vi "Set Maximum Data Length.vi"(9 "maximum data length":i32=-1, 11 "variant in":variant) -> (3 "variant out":variant)   [LabVIEW 2017]
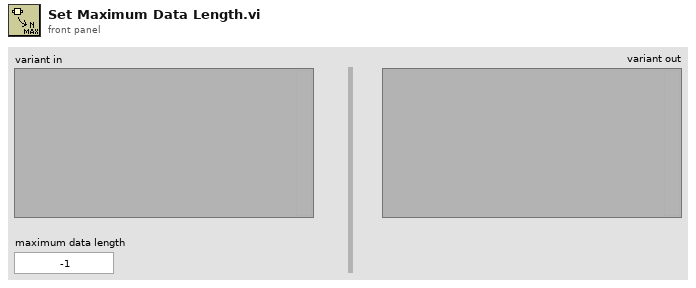
[diagram p1: front panel]
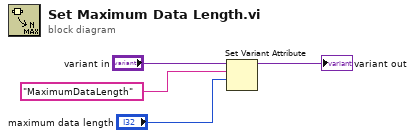
[diagram p0: block diagram]
diagram:
  n1 = Set Variant Attribute(Variant="variant in", name="MaximumDataLength", value="maximum data length") -> (Variant out=→"variant out":variant)  [unwired: 1 in, 2 out]
